vi "generateimagejmacro.vi"(7 "file format":T1, 8 "number of recorded frames":i16, 11 "Reso or Galvo?":bool=TRUE) -> ()   [LabVIEW 2012]
doc: "SciScan 1.2 160622"
uses:
  Custom Controls/file format type def.ctl
  GFG/GFGpathGet.vi
  GFG/GFGnumericGet.vi
  GFG/GFGbooleanGet.vi
  GFG/GFG library.lvlib
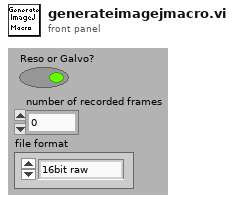
[diagram p1: front panel]
types:
  T1 = typedef "file format type def.ctl" = enum16{"16bit raw", "32bit raw", "16bit multi-tiff (interleave)", "16bit multi-tiff (separate)", "16bit multi-tiff (stacked)", "32bit multi-tiff (interleave)", "32bit multi-tiff (separate)", "32bit multi-tiff (stacked)", "16bit tiff series (interleave)", "16bit tiff series (separate)", "16bit tiff series (stacked)", "32bit tiff series (interleave)", "32bit tiff series (separate)", "32bit tiff series (stacked)"}
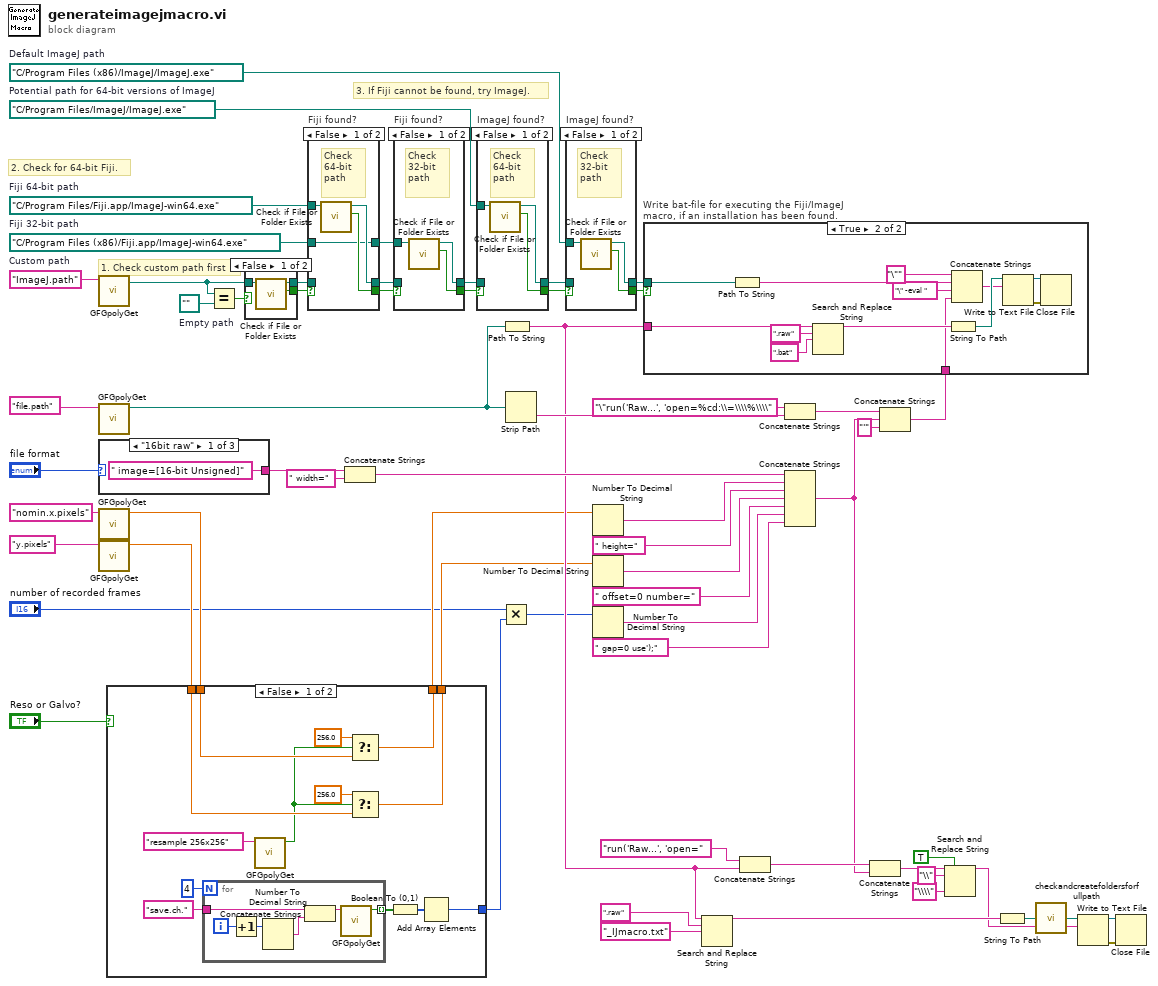
[diagram p0: block diagram]
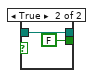
[diagram p2: hidden frame]
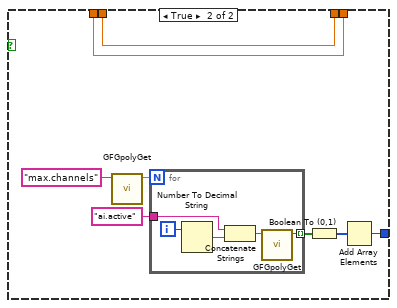
[diagram p7: hidden frame]
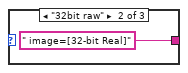
[diagram p9: hidden frame]
diagram:
  w3 = path ""  # Empty path
  w14 = path "C:/Program Files/Fiji.app/ImageJ-win64.exe"  # Fiji 64-bit path
  w15 = path "C:/Program Files (x86)/Fiji.app/ImageJ-win64.exe"  # Fiji 32-bit path
  w9 = path "C:/Program Files/ImageJ/ImageJ.exe"  # Potential path for 64-bit versions of ImageJ
  w8 = path "C:/Program Files (x86)/ImageJ/ImageJ.exe"  # Default ImageJ path
  w31 = "ImageJ.path"  # Custom path
  # "2. Check for 64-bit Fiji."
  # "3. If Fiji cannot be found, try ImageJ."
  # "1. Check custom path first"
  n1 = call-poly "GFGpolyGet.vi"("Variable Name in"=w31) -> ("Path"=w2:path)  [unwired: 8 in, 2 out]
  n2 = call-poly "GFGpolyGet.vi"("Variable Name in"="file.path" ("Tag in")) -> ("Path"=w36:path)  [unwired: 8 in, 2 out]
  n3 = case shown="\"16bit raw\"" "file format" {
    tunnel: [" image=[16-bit Unsigned]" ("image type") " image=[32-bit Real]" ("image type") _] -> w34
    frame "16bit raw" {
    }
    frame "32bit raw" {
    }
    frame Default {
    }
  }
  n4 = call-poly "GFGpolyGet.vi"("Variable Name in"="nomin.x.pixels") -> ("Numeric"=w24:dbl)  [unwired: 8 in, 2 out]
  n5 = call-poly "GFGpolyGet.vi"("Variable Name in"="y.pixels") -> ("Numeric"=w26:dbl)  [unwired: 8 in, 2 out]
  n6 = case shown="False" "Reso or Galvo?" {
    tunnel: [w66 w86] -> w32
    tunnel: [w70 w85] -> w25
    tunnel: w26 -> [w72 w85]
    tunnel: [w73 w84] -> w23
    tunnel: w24 -> [w74 w84]
    frame False {
      n7 = for {
        N: 4 -> [_]
        tunnel: "save.ch." ("Variable Name in") -> [w83]
        tunnel: [w82] -> w68 mode=indexing
        i -> [w81]
        n8 = Increment(x=w81) -> (x+1=w80:i32)
        n9 = Number To Decimal String(number=w80) -> (decimal integer string=w78:string)  [unwired: 1 in]
        n10 = Concatenate Strings(w83, w78) -> (w79:string)
        n11 = call-poly "GFGpolyGet.vi"("Variable Name in"=w79) -> ("Boolean Value OUT"=w82:bool)  [unwired: 9 in, 1 out]
      }
      n12 = call-poly "GFGpolyGet.vi"("Variable Name in"="resample 256x256") -> ("Boolean Value OUT"=w71:bool)  [unwired: 9 in, 1 out]
      n13 = Select(t=256.0, s=w71, f=w74) -> (s? t:f=w73:dbl)
      n14 = Select(t=256.0, s=w71, f=w72) -> (s? t:f=w70:dbl)
      n15 = Boolean To (0,1)(Boolean=w68) -> (0, 1=w67:i16[])
      n16 = Add Array Elements(numeric array=w67) -> (sum=w66:i16)
    }
    frame True {
      n17 = call-poly "GFGpolyGet.vi"("Variable Name in"="max.channels") -> ("Numeric"=w90:dbl)  [unwired: 8 in, 2 out]
      n18 = for {
        N: w90 -> [_]
        tunnel: [w96] -> w88 mode=indexing
        tunnel: "ai.active" ("Variable Name in") -> [w95]
        i -> [w94]
        n19 = Number To Decimal String(number=w94) -> (decimal integer string=w93:string)  [unwired: 1 in]
        n20 = Concatenate Strings(w95, w93) -> (w92:string)
        n21 = call-poly "GFGpolyGet.vi"("Variable Name in"=w92) -> ("Boolean Value OUT"=w96:bool)  [unwired: 9 in, 1 out]
      }
      n22 = Boolean To (0,1)(Boolean=w88) -> (0, 1=w87:i16[])
      n23 = Add Array Elements(numeric array=w87) -> (sum=w86:i16)
    }
  }
  n24 = Equal?(x=w2, y=w3) -> (x = y?=w1:bool)
  n25 = case shown="False" w1 {
    tunnel: [w99 FALSE ("file or folder exists?")] -> w20
    tunnel: [w98 w100] -> w19
    tunnel: w2 -> [w97 w100]
    frame False {
      n26 = call <vilib>:"Check if File or Folder Exists.vi"("path"=w97) -> ("file or folder exists?"=w99:bool, "dup path"=w98:path)  [unwired: 8 in, 1 out]
    }
    frame True {
    }
  }
  n27 = case "Fiji found?" shown="False" w20 {
    selector: w20 -> [_ w107]
    tunnel: w19 -> [_ w108]
    tunnel: [w103 w108] -> w17
    tunnel: [w104 w107] -> w18
    tunnel: w15 -> [w102 w106]
    tunnel: w14 -> [w105 _]
    tunnel: [w102 w106] -> w16
    frame False {
      # "Check 64-bit path"
      n28 = call <vilib>:"Check if File or Folder Exists.vi"("path"=w105) -> ("file or folder exists?"=w104:bool, "dup path"=w103:path)  [unwired: 8 in, 1 out]
    }
    frame True {
    }
  }
  n29 = Concatenate Strings(w34, " width=" ("string")) -> (w55:string)
  n30 = case "Fiji found?" shown="False" w18 {
    selector: w18 -> [_ w112]
    tunnel: [w110 w112] -> w10
    tunnel: w17 -> [_ w113]
    tunnel: [w109 w113] -> w11
    tunnel: w16 -> [w111 _]
    frame False {
      # "Check 32-bit path"
      n31 = call <vilib>:"Check if File or Folder Exists.vi"("path"=w111) -> ("file or folder exists?"=w110:bool, "dup path"=w109:path)  [unwired: 8 in, 1 out]
    }
    frame True {
    }
  }
  n32 = case "ImageJ found?" shown="False" w10 {
    selector: w10 -> [_ w117]
    tunnel: w11 -> [_ w118]
    tunnel: [w114 w118] -> w13
    tunnel: [w115 w117] -> w12
    tunnel: w9 -> [w116 _]
    frame False {
      # "Check 64-bit path"
      n33 = call <vilib>:"Check if File or Folder Exists.vi"("path"=w116) -> ("file or folder exists?"=w115:bool, "dup path"=w114:path)  [unwired: 8 in, 1 out]
    }
    frame True {
    }
  }
  n34 = Multiply(x="number of recorded frames", y=w32) -> (x*y=w28:i16)
  n35 = Path To String(path=w36) -> (string=w44:string)
  n36 = Strip Path(path=w36) -> (name=w53:string)  [unwired: 1 out]
  n37 = case "ImageJ found?" shown="False" w12 {
    selector: w12 -> [_ w122]
    tunnel: [w120 w122] -> w6
    tunnel: w13 -> [_ w123]
    tunnel: [w119 w123] -> w7
    tunnel: w8 -> [w121 _]
    frame False {
      # "Check 32-bit path"
      n38 = call <vilib>:"Check if File or Folder Exists.vi"("path"=w121) -> ("file or folder exists?"=w120:bool, "dup path"=w119:path)  [unwired: 8 in, 1 out]
    }
    frame True {
    }
  }
  n39 = Number To Decimal String(number=w23) -> (decimal integer string=w62:string)  [unwired: 1 in]
  n40 = Number To Decimal String(number=w25) -> (decimal integer string=w60:string)  [unwired: 1 in]
  n41 = Number To Decimal String(number=w28) -> (decimal integer string=w58:string)  [unwired: 1 in]
  n42 = Search and Replace String(input string=w44, search string=".raw", replace string="_IJmacro.txt" ("string")) -> (result string=w39:string)  [unwired: 5 in, 3 out]
  n43 = Concatenate Strings("run('Raw...', 'open=", w44) -> (w48:string)
  n44 = Concatenate Strings("\"run('Raw...', 'open=%cd:\\=\\\\%\\\\", w53) -> (w52:string)
  n45 = Concatenate Strings(w55, w62, " height=", w60, " offset=0 number=", w58, " gap=0 use');") -> (w47:string)
  n46 = Concatenate Strings(w48, w47) -> (w40:string)
  n47 = Concatenate Strings(w52, w47, "'" ("string")) -> (w50:string)
  n48 = case "Write bat-file for executing the Fiji/ImageJ macro, if an installation has been found." shown="True" w6 {
    tunnel: w50 -> [_ w130]
    tunnel: w44 -> [_ w129]
    tunnel: w7 -> [_ w128]
    frame False {
    }
    frame True {
      n49 = Path To String(path=w128) -> (string=w127:string)
      n50 = Search and Replace String(input string=w129, search string=".raw", replace string=".bat" ("string")) -> (result string=w132:string)  [unwired: 5 in, 3 out]
      n51 = String To Path(string=w132) -> (path=w133:path)
      n52 = Concatenate Strings("\"" ("string"), w127, "\" -eval " ("string"), w130) -> (w131:string)
      n53 = Write to Text File(file (use dialog)=w133, text=w131) -> (refnum out=w125:refnum<file>, error out=w124:errorcluster)  [unwired: 2 in, 1 out]
      n54 = Close File(refnum=w125, error in=w124) -> ()  [unwired: 2 out]
    }
  }
  n55 = Search and Replace String(replace all?=TRUE ("replace all? (F)"), input string=w40, search string="\\", replace string="\\\\" ("replace string (\"\")")) -> (result string=w38:string)  [unwired: 4 in, 3 out]
  n56 = String To Path(string=w39) -> (path=w30:path)
  n57 = call "checkandcreatefoldersforfullpath.vi"("Path IN"=w30) -> ("Path OUT"=w29:path)  [unwired: 4 in]
  n58 = Write to Text File(file (use dialog)=w29, text=w38) -> (refnum out=w5:refnum<file>, error out=w4:errorcluster)  [unwired: 2 in, 1 out]
  n59 = Close File(refnum=w5, error in=w4) -> ()  [unwired: 2 out]
